vi "Command (read & write) - AM.vi"(7 "timeout ms (100)":i32=100, 8 "error in (no error)":errorcluster, 9 "Max. Acceleration":dbl=-9999.0, 10 "IP":string, 11 "connection ID in":refnum<k16>) -> (0 "error out":errorcluster, 3 "connection ID out":refnum<k16>)   [LabVIEW 2016, in "SMD-7615.lvlib" / "eSCL.lvlib"]
doc: "AM - Max Acceleration\nSets or requests the maximum acceleration/deceleration allowed when using analog velocity and oscillator modes. Also sets the deceleration rate used when an end-of-travel limit is activated during a move or when an ST (Stop) or SK (Stop & Kill) command is sent.\nParameter:\nAM - request max. Accelerarion\nAM200 Set maximum acceleration/deceleration to 200rev/sec/sec"
uses:
  eSCL.lvlib
  DBL Command and Param.ctl
panel:
  out "max acceleration":dbl
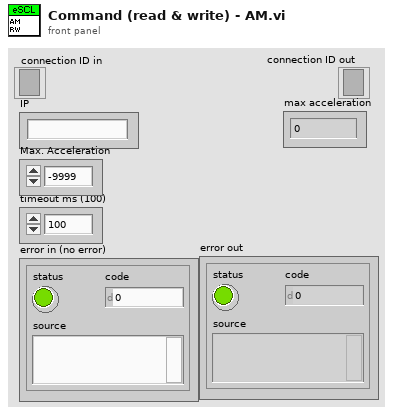
[diagram p1: front panel]
types:
  T1 = typedef "SMD-7615.lvlib/eSCL.lvlib/DBL Command and Param.ctl" = cluster{"Command":string, "DBL Parameler":dbl, "DBL Parameler Default":dbl, "DBL Parameler Coerece Upper":dbl, "DBL Parameler Coerece Lower":dbl}
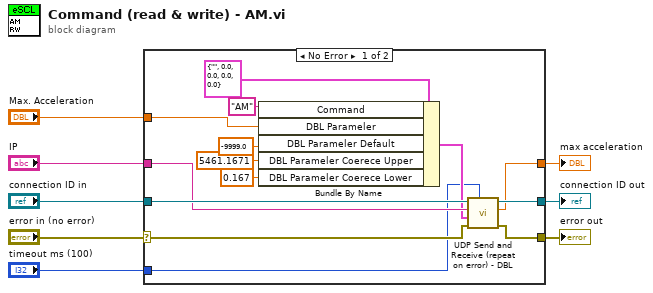
[diagram p0: block diagram]
diagram:
  n1 = case shown="No Error" "error in (no error)" {
    selector: "error in (no error)" -> [w13 w23]
    tunnel: "connection ID in" -> [w16 w24]
    tunnel: [w11 w24] -> w2
    tunnel: [w10 w23] -> w1
    tunnel: "IP" -> [w15 _]
    tunnel: "timeout ms (100)" -> [w12 _]
    tunnel: [w9 _] -> w3
    tunnel: "Max. Acceleration" -> [w17 _]
    frame No Error {
      n2 = Bundle By Name(cluster=T1 {"Command"="", "DBL Parameler"=0.0, "DBL Parameler Default"=0.0, "DBL Parameler Coerece Upper"=0.0, "DBL Parameler Coerece Lower"=0.0} ("DBL Command & Param"), "Command"="AM", "DBL Parameler"=w17, "DBL Parameler Default"=-9999.0, "DBL Parameler Coerece Upper"=5461.1671, "DBL Parameler Coerece Lower"=0.167) -> (w14:T1)
      n3 = call "UDP Send and Receive (repeat on error) - DBL.vi"("timeout ms (100)"=w12, "error in (no error)"=w13, "DBL Command & Param"=w14, "IP"=w15, "connection ID in"=w16) -> ("error out"=w10:errorcluster, "DBL Param out"=w9:dbl, "connection ID out"=w11:refnum<k16>)  [unwired: 4 in]
    }
    frame Error {
    }
  }
  "connection ID out" <- w2
  "error out" <- w1
  "max acceleration" <- w3
